vi "AlliGator Get-Set Phasor Color Map Vertices.vi"(8 "Set/Get(F)":bool, 9 "Decay Range Exponent in":dbl, 10 "Color Array in":u32[](array[colorbox]), 11 "Vertices in":cluster{"X":dbl, "Y":dbl}[](array[cluster])) -> (0 "Empty?":bool, 1 "Decay Range Exponent out":dbl, 2 "Color Array out":u32[](array[colorbox]), 3 "Vertices out":cluster{"X":dbl, "Y":dbl}[](array[cluster]))   [LabVIEW 2021, in "AlliGator Phasor Plot Color Map.lvlib"]
doc: "Stores color map vertices and their colors."
uses:
  AlliGator Phasor Plot Color Map.lvlib
panel:
  # "see the AlliGator License on the block diagram (Ctrl+E or Window:Show Block Diagram)"
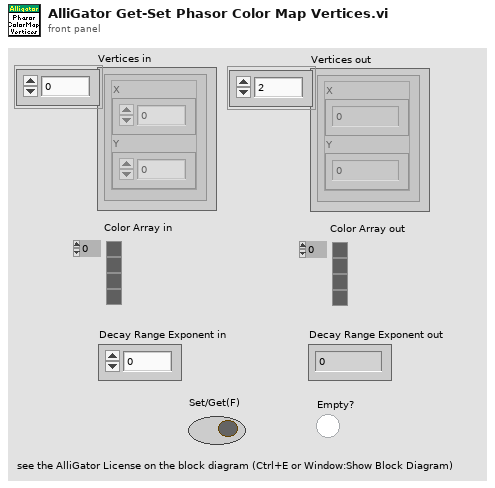
[diagram p1: front panel]
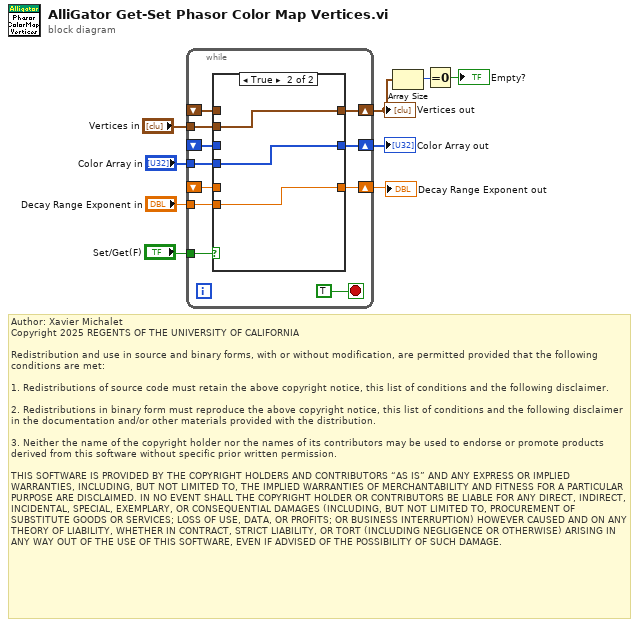
[diagram p0: block diagram]
diagram:
  # "Author: Xavier Michalet\nCopyright 2025 REGENTS OF THE UNIVERSITY OF CALIFORNIA\n\nRedistribution and use in source and binary forms, with or without modification, are permitted provided that the following conditions are met:\n\n1. Redistributions of source code must retain the above copyright notice, this list of conditions and the following disclaimer.\n\n2. Redistributions in binary form must reproduce the above copyright notice, this list of conditions and the following disclaimer in the documentation and/or other materials provided with the distribution.\n\n3. Neither the name of the copyright holder nor the names of its contributors may be used to endorse or promote products derived from this software without specific prior written permission.\n\nTHIS SOFTWARE IS PROVIDED BY THE COPYRIGHT HOLDERS AND CONTRIBUTORS “AS IS” AND ANY EXPRESS OR IMPLIED WARRANTIES, INCLUDING, BUT NOT LIMITED TO, THE IMPLIED WARRANTIES OF MERCHANTABILITY AND FITNESS FOR A PARTICULAR PURPOSE ARE DISCLAIMED. IN NO EVENT SHALL THE COPYRIGHT HOLDER OR CONTRIBUTORS BE LIABLE FOR ANY DIRECT, INDIRECT, INCIDENTAL, SPECIAL, EXEMPLARY, OR CONSEQUENTIAL DAMAGES (INCLUDING, BUT NOT LIMITED TO, PROCUREMENT OF SUBSTITUTE GOODS OR SERVICES; LOSS OF USE, DATA, OR PROFITS; OR BUSINESS INTERRUPTION) HOWEVER CAUSED AND ON ANY THEORY OF LIABILITY, WHETHER IN CONTRACT, STRICT LIABILITY, OR TORT (INCLUDING NEGLIGENCE OR OTHERWISE) ARISING IN ANY WAY OUT OF THE USE OF THIS SOFTWARE, EVEN IF ADVISED OF THE POSSIBILITY OF SUCH DAMAGE."
  n1 = while {
    tunnel: "Set/Get(F)" -> [w20]
    shift-right: [w18] -> w3
    shift-left: _ -> [w16]
    tunnel: "Vertices in" -> [w19]
    shift-right: [w15] -> w6
    shift-left: _ -> [w13]
    tunnel: "Color Array in" -> [w14]
    shift-right: [w12] -> w5
    shift-left: _ -> [w10]
    tunnel: "Decay Range Exponent in" -> [w11]
    stop <- TRUE stop-if-true
    n2 = case shown="True" w20 {
      tunnel: w19 -> [_ w26]
      tunnel: [w23 w26] -> w18
      tunnel: w16 -> [w23 _]
      tunnel: [w22 w25] -> w15
      tunnel: w14 -> [_ w25]
      tunnel: w13 -> [w22 _]
      tunnel: [w21 w24] -> w12
      tunnel: w11 -> [_ w24]
      tunnel: w10 -> [w21 _]
      frame False {
      }
      frame True {
      }
    }
  }
  "Vertices out" <- w3
  "Color Array out" <- w6
  "Decay Range Exponent out" <- w5
  n3 = Array Size(array=w3) -> (size(s)=w2:i32)
  n4 = Equal To 0?(x=w2) -> (x = 0?=→"Empty?":bool)
